vi "Climb Loop.vi"   [LabVIEW 2017]
uses:
  Robot Global Data.vi
  <vilib>/Rock Robotics/WPI/Solenoid/Deprecated/WPI_SolenoidSetBool.vi
types:
  T1 = typedef "Climb Command Cluster.ctl" = cluster{"Climb":bool}
  T2 = typedef "WPI_SolenoidDevRef.ctl" = cluster{"DevStatus":errorcluster, "Pneumatics Control Module":u8, "Forward Solenoid Channel":T3, "Reverse Solenoid Channel":T3}
  T3 = typedef "WPI_SolenoidChannel.ctl" = enum8{"Solenoid 0", "Solenoid 1", "Solenoid 2", "Solenoid 3", "Solenoid 4", "Solenoid 5", "Solenoid 6", "Solenoid 7", "Invalid"}
  T4 = typedef "Climb Status Cluster.ctl" = cluster{"Climb":bool, "Time Remaining":dbl}
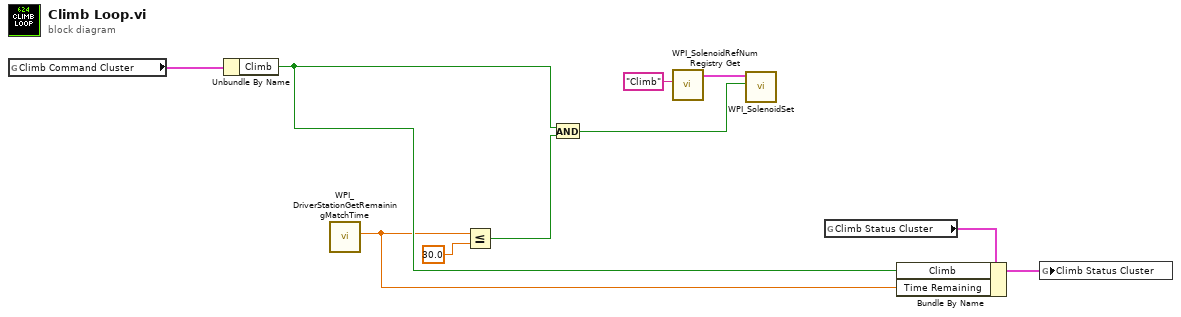
[diagram p0: block diagram]
diagram:
  n1 = global read "Robot Global Data.vi" "Climb Command Cluster"() -> (w10:T1)
  n2 = Unbundle By Name(w10) -> ("Climb"=w6:bool)
  n3 = call <vilib>:"WPI_DriverStationGetRemainingMatchTime.vi"() -> ("Match Time(s)"=w2:sgl)  [unwired: 10 in, 1 out]
  n4 = Less Or Equal?(x=w2, y=30.0) -> (x <= y?=w7:bool)
  n5 = And(x=w6, y=w7) -> (x .and. y?=w3:bool)
  n6 = call <vilib>:"WPI_SolenoidRefNum Registry Get.vi"("refnum name"="Climb") -> ("SolenoidDevRef"=w4:T2)  [unwired: 9 in, 1 out]
  n7 = call-poly <vilib>:"WPI_SolenoidSet.vi"("Value"=w3, "SolenoidDevRef"=w4) -> ()  [unwired: 8 in, 2 out]
  n8 = global read "Robot Global Data.vi" "Climb Status Cluster"() -> (w1:T4)
  n9 = Bundle By Name(cluster=w1, "Climb"=w6, "Time Remaining"=w2) -> (w9:T4)
  n10 = global write "Robot Global Data.vi" "Climb Status Cluster"(w9) -> ()
